vi "RT Loop - Acquire camera_test_1.vi"(11 "Camera Queue  in":refnum<k33>) -> (0 "error out":errorcluster)   [LabVIEW 2017]
uses:
  <vilib>/vision/Image Controls.llb/IMAQ Image.ctl
  <vilib>/userdefined/High Color/IMAQdx.ctl
  <vilib>/vision/driver/NI_Vision_Acquisition_Software.lvlib
panel:
  in  "Boolean":bool
  out "empty? 2":bool
  in  "y":bool
  out "Webcam":T1(plugin-control)
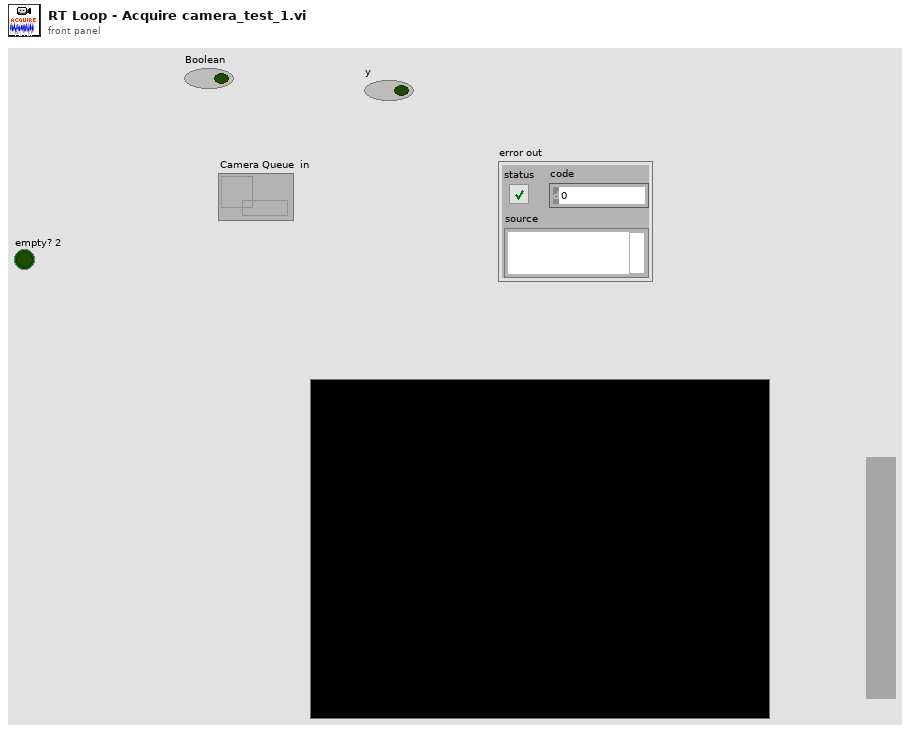
[diagram p1: front panel]
types:
  T1 = typedef "IMAQ Image.ctl" = refnum<image>
  T2 = typedef "IMAQdx.ctl" = refnum<k21>
  T3 = typedef "Image Type" = u32
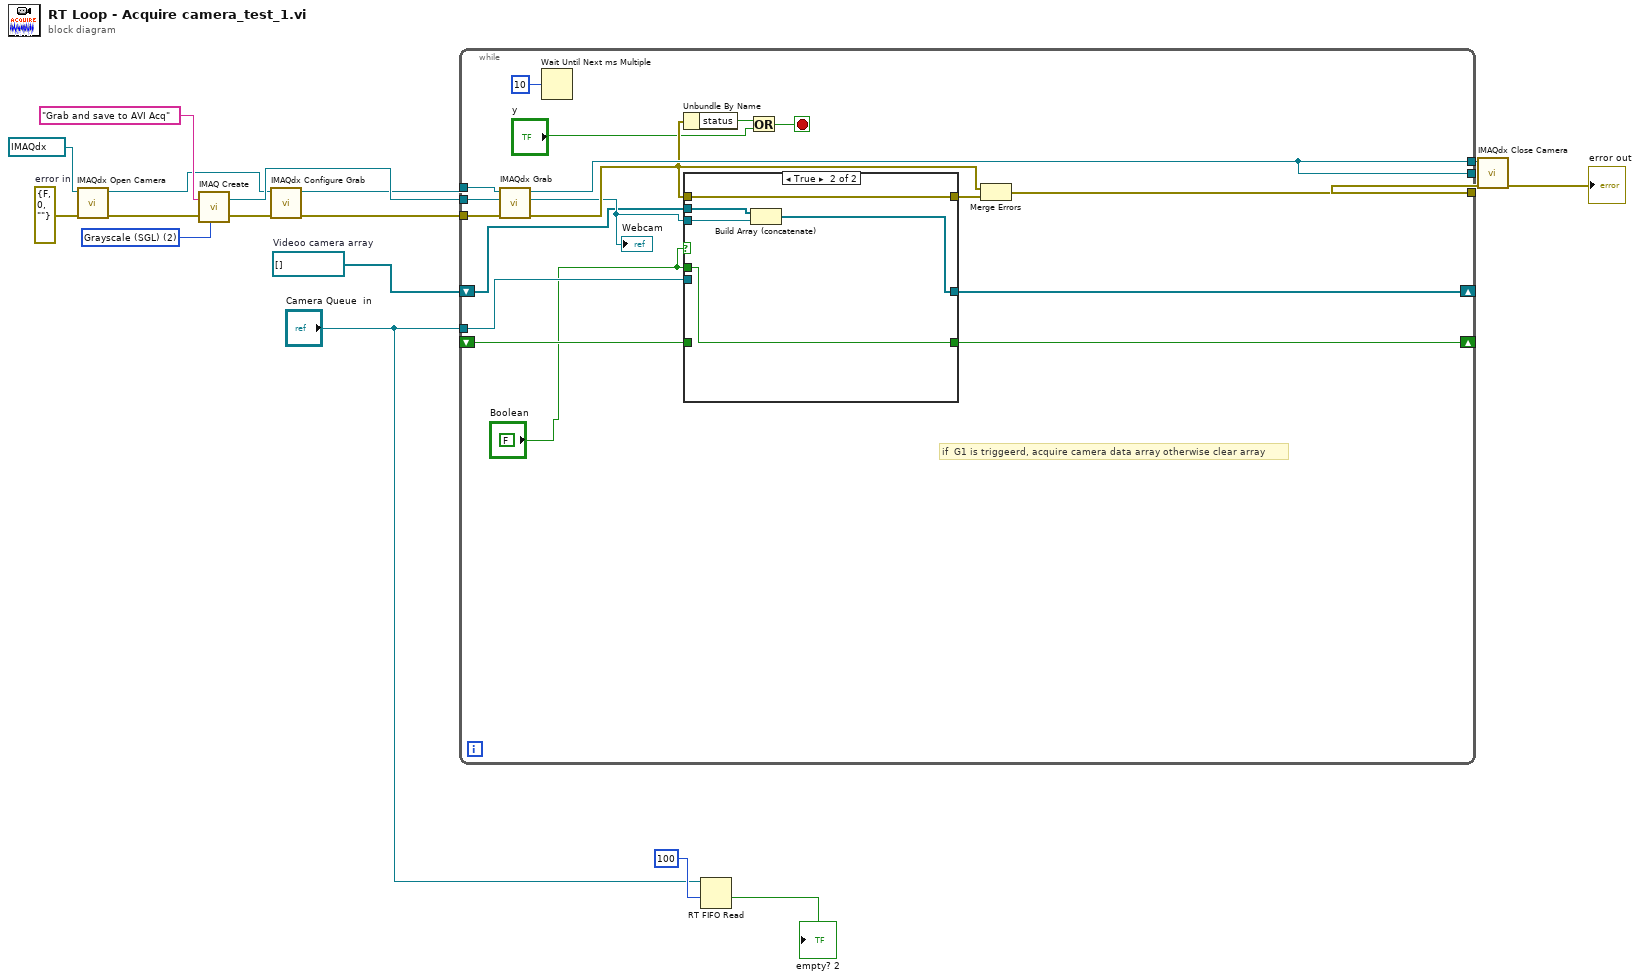
[diagram p0: block diagram]
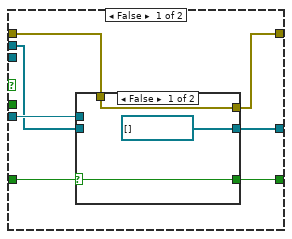
[diagram p2: hidden frame]
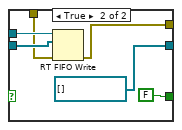
[diagram p3: hidden frame]
diagram:
  w4 = T1[] []  # Videoo camera array
  w10 = T3 2 items=["Grayscale (U8)", "Grayscale (I16)", "Grayscale (SGL)", "Complex (CSG)", "RGB (U32)", "HSL (U32)", "RGB (U64)", "Grayscale (U16)"] ("Image Type")
  w8 = errorcluster {"status"=FALSE, "code"=0, "source"=""}  # error in
  n1 = call <vilib>:"IMAQdx Open Camera.vi"("error in"=w8, "Session In"=T2 "cam0") -> ("error out"=w11:errorcluster, "Session Out"=w6:T2)  [unwired: 8 in]
  n2 = call "IMAQ Create"("Image Name"="Grab and save to AVI Acq", "Image Type"=w10, "error in (no error)"=w11) -> ("New Image"=w13:T1, "error out"=w14:errorcluster)  [unwired: 2 in]
  n3 = call <vilib>:"IMAQdx Configure Grab.vi"("error in"=w14, "Session In"=w6) -> ("error out"=w15:errorcluster, "Session Out"=w12:T2)  [unwired: 8 in]
  n4 = while {
    tunnel: [w29] -> _
    shift-right: [w28] -> _
    shift-left: w4 -> [w21]
    tunnel: "Camera Queue  in" -> [w19]
    tunnel: w12 -> [w33]
    tunnel: w13 -> [w32]
    tunnel: w15 -> [w31]
    tunnel: [w29] -> w16
    tunnel: [w25] -> w5
    shift-right: [w23] -> _
    shift-left: _ -> [w22]
    stop <- w30 stop-if-true
    (unwired) FALSE ("Boolean")
    # "if  G1 is triggeerd, acquire camera data array otherwise clear array"
    n5 = call <vilib>:"IMAQdx Grab.vi"("error in"=w31, "Image In"=w32, "Session In"=w33) -> ("error out"=w26:errorcluster, "Image Out"=w24:T1, "Session Out"=w29:T2)  [unwired: 5 in, 1 out]
    "Webcam" <- w24
    n6 = Wait Until Next ms Multiple(millisecond multiple=u32 10 ("milliseconds to wait")) -> ()  [unwired: 1 out]
    n7 = Unbundle By Name(w26) -> ("status"=w34:bool)
    n8 = case shown="True" "Boolean" {
      tunnel: [w39 w53] -> w28
      tunnel: w19 -> [w40 _]
      tunnel: w26 -> [w37 w56]
      tunnel: [w36 w56] -> w27
      tunnel: w21 -> [w38 w55]
      tunnel: w24 -> [_ w54]
      tunnel: [w41 w52] -> w23
      tunnel: "Boolean" -> [_ w52]
      tunnel: w22 -> [w42 _]
      frame False {
        n9 = case shown="False" w42 {
          selector: w42 -> [w45 _]
          tunnel: [w45 FALSE] -> w41
          tunnel: w40 -> [_ w50]
          tunnel: w38 -> [_ w48]
          tunnel: [T1[] [] T1[] []] -> w39
          tunnel: w37 -> [w43 w47]
          tunnel: [w43 w46] -> w36
          frame False {
          }
          frame True {
            n10 = RT FIFO Write(0:w50, 1:w48, 3:w47) -> (11:w46:errorcluster)  [unwired: 2 in, 3 out]
          }
        }
      }
      frame True {
        n11 = Build Array (concatenate)(w55, w54) -> (w53:T1[])
      }
    }
    n12 = Or(x=w34, y="y") -> (x .or. y?=w30:bool)
    n13 = Merge Errors(w26, w27) -> (w25:errorcluster)
  }
  n14 = RT FIFO Read(0:"Camera Queue  in", 2:100 ("ms timeout (0)")) -> (10:→"empty? 2":bool)  [unwired: 2 in, 4 out]
  n15 = call <vilib>:"IMAQdx Close Camera.vi"("error in"=w5, "Session In"=w16) -> ("error out"=→"error out":errorcluster)  [unwired: 9 in]
